vi "Report.vi"() -> ()   [LabVIEW 2017]
uses:
  <vilib>/Utility/miscctls.llb/LVRowAndColumnUnsignedTypeDef.ctl
  bcf87072-937c-4590-92ea-1cc62e0fba93.vi
  a160b8e7-0040-4e34-a052-5f80b3aab475.vi
  <vilib>/Array/Sort 2D Array - Pop Stack.vi
  <vilib>/Array/Sort 2D Array - Push Stack.vi
  <vilib>/addons/database/Connection.llb/DB Tools Open Connec (String).vi
  <vilib>/addons/database/Auxilliary.llb/DB Tools Format Datetime String (Time Stamp).vi
  <vilib>/Utility/file.llb/Write Delimited Spreadsheet (string).vi
  Global/Global 1.vi
  <vilib>/regexp/Match Regular Expression.xnode
  <vilib>/addons/database/NI_Database_API.lvlib
  <vilib>/Utility/NIReport.llb/NI_report.lvclass
  <vilib>/Utility/NIReport.llb/Append Text Table to Report (wrap).vi
panel:
  out "to date/time":string
  out "from date/time":string
  out "reposr save header":string[](array[string])
  in  "SELECT REPORT TYPE":string(combo)="WITH TRECIABILITY"
  out "error out":errorcluster
  in  "error in (no error)":errorcluster
  in  "GET REPORT":bool
  in  "EXIT":bool
  in  "EXPORT TO EXCEL":bool
  in  "TO":timestamp format="%<%x>T"
  in  "FROM":timestamp format="%<%x>T"
  in  "BARCODE":string
  in  "TYPE":string(combo)="DATE TIME"
  in  "STATION WISE":string(combo)="0"
  out "Table":string[][](table)
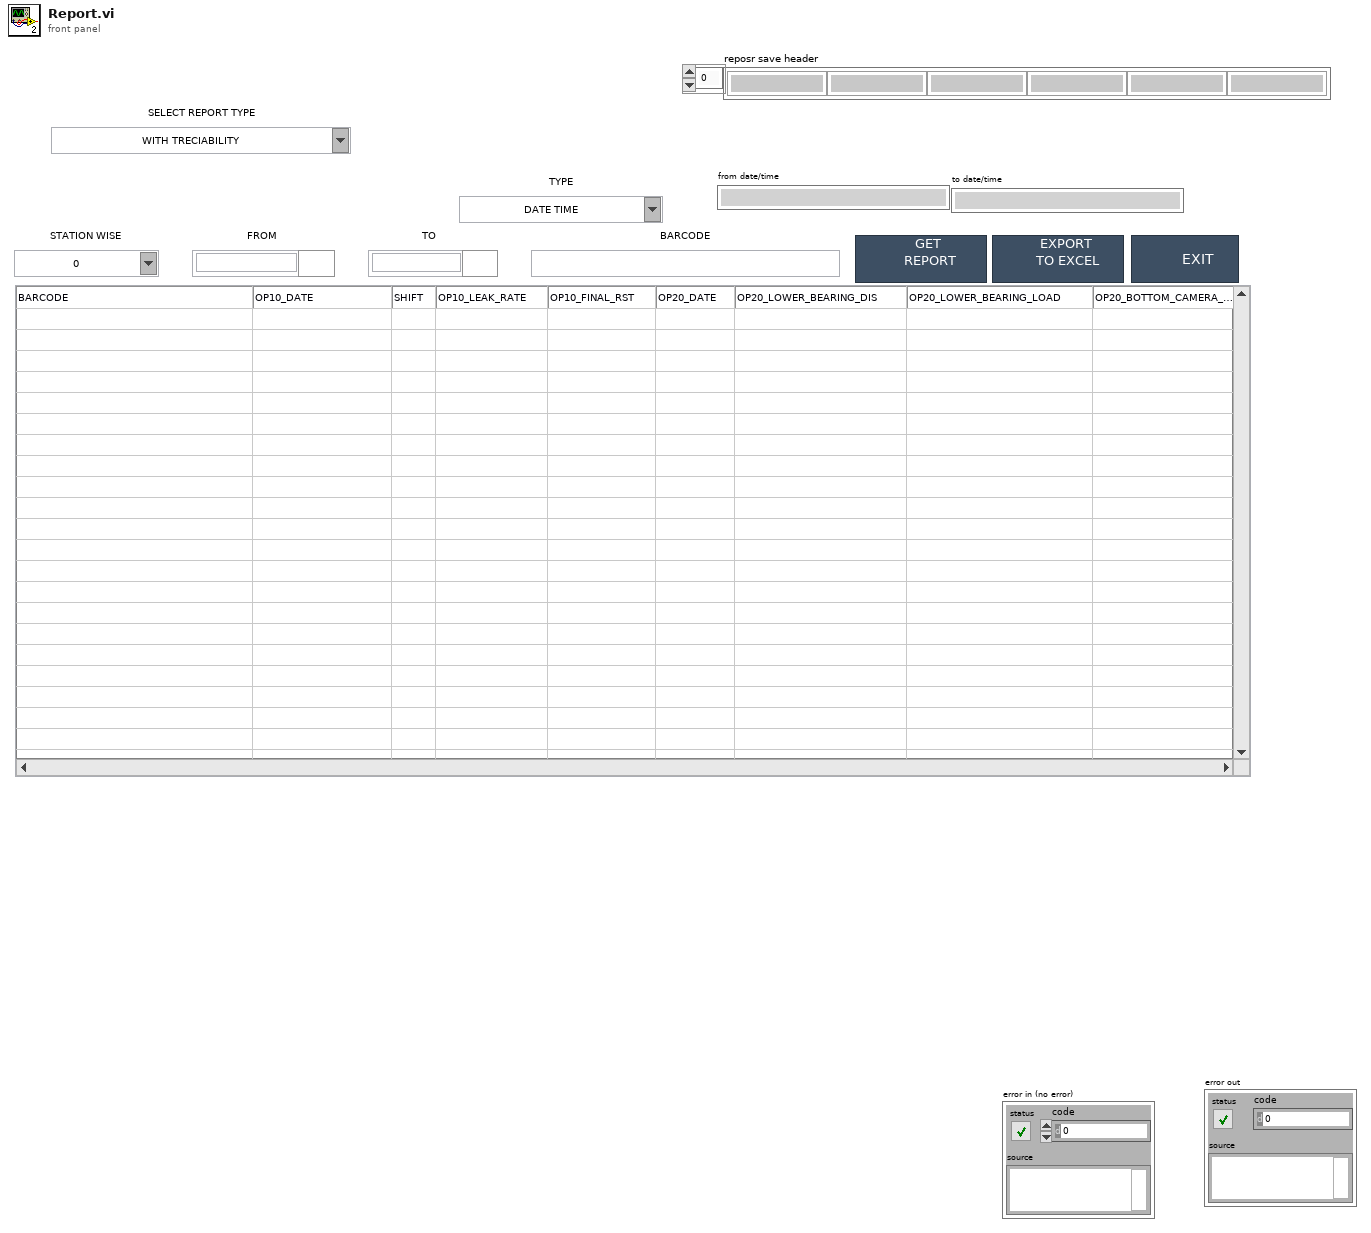
[diagram p1: front panel]
types:
  T1 = typedef "NI_Database_API.lvlib/Conn ObjectReference.ctl" = refnum<k1>
  T2 = typedef "LVRowAndColumnUnsignedTypeDef.ctl" = cluster{"Row":u32, "Column":u32}
  T3 = enum16{"Standard Report", "HTML", "Word", "Excel"}
  T4 = enum16{"maximized", "minimized", "normal", "no change"}
  T5 = typedef "LVRowAndColumnTypeDef.ctl" = cluster{"Row":i32, "Column":i32}
  T6 = enum32{"invalid app kind", "Development System", "Run Time System", "Student Edition", "Embedded LabVIEW", "Evaluation", "Custom"}
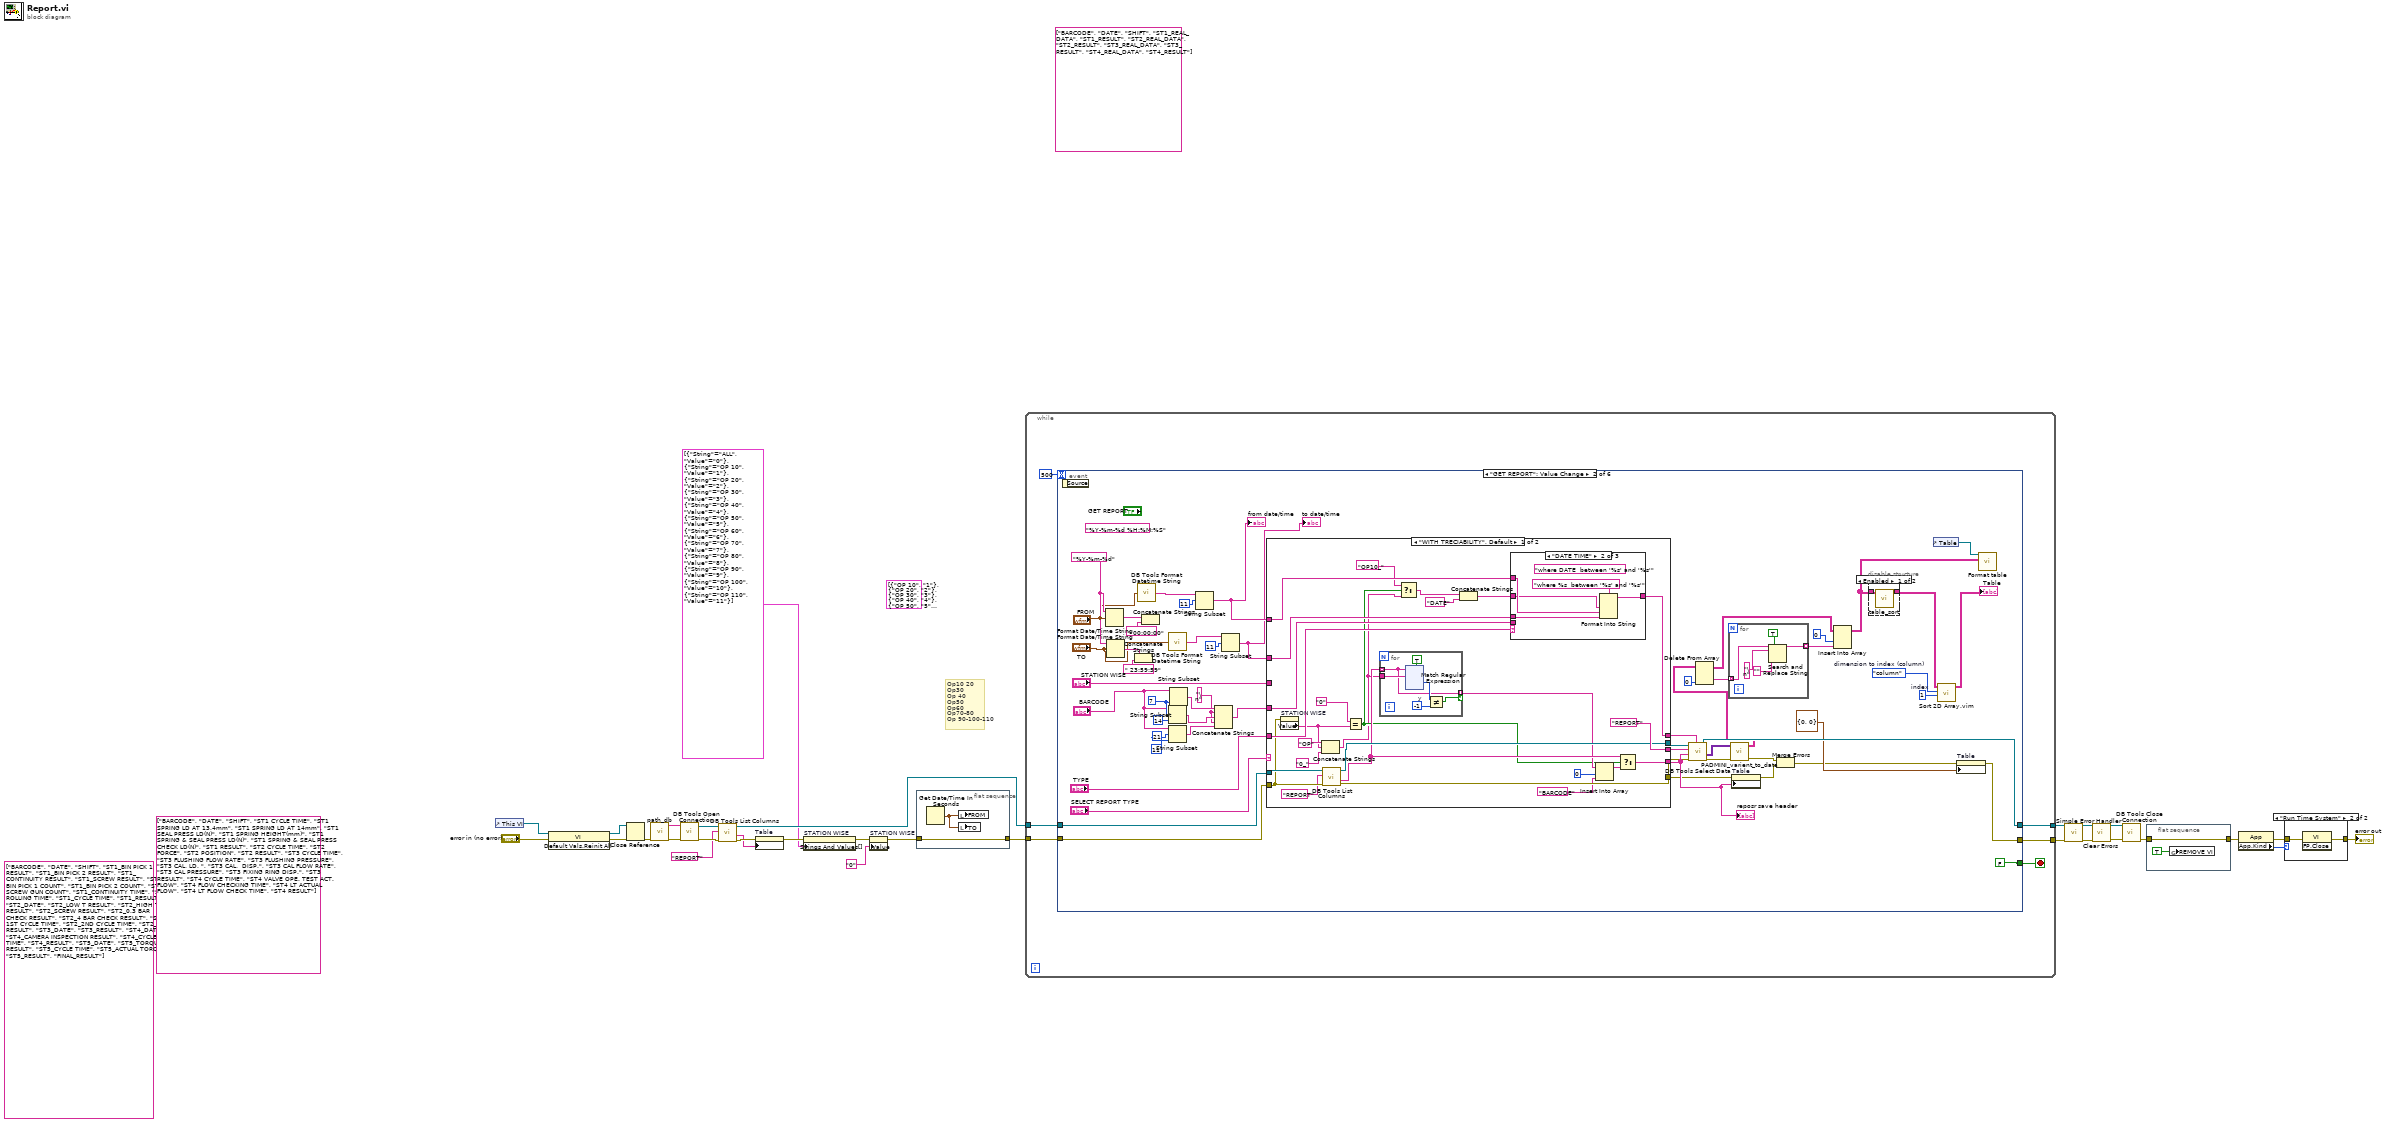
[diagram p0: block diagram]
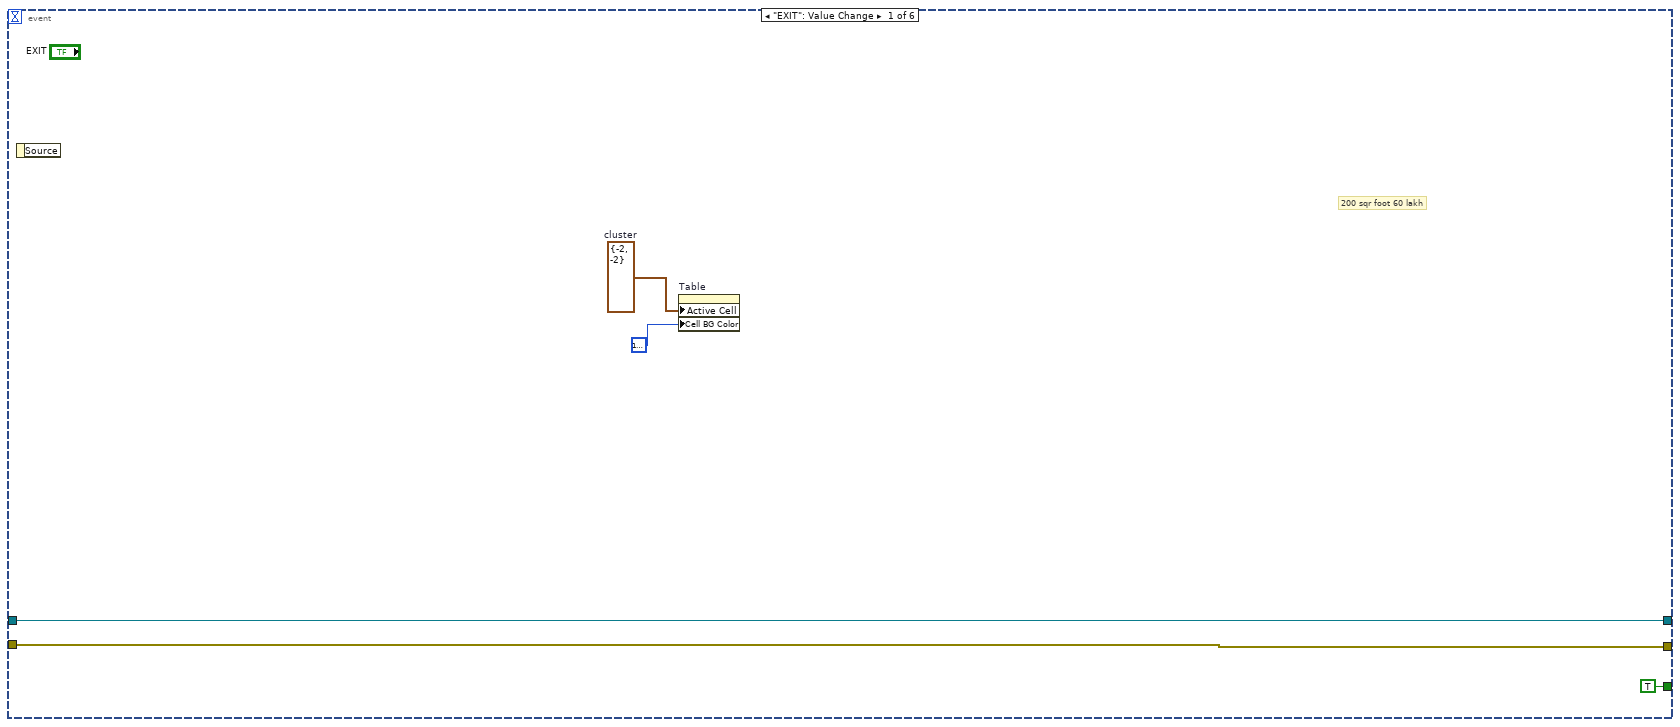
[diagram p2: hidden frame]
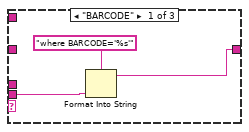
[diagram p4: hidden frame]
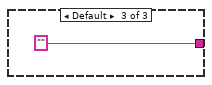
[diagram p5: hidden frame]
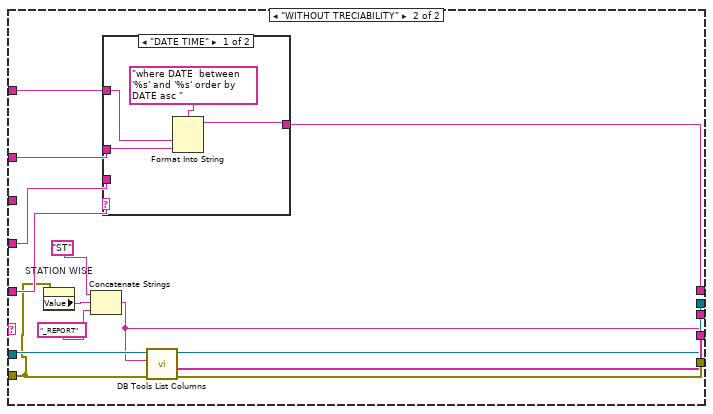
[diagram p6: hidden frame]
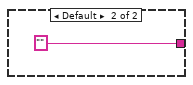
[diagram p7: hidden frame]
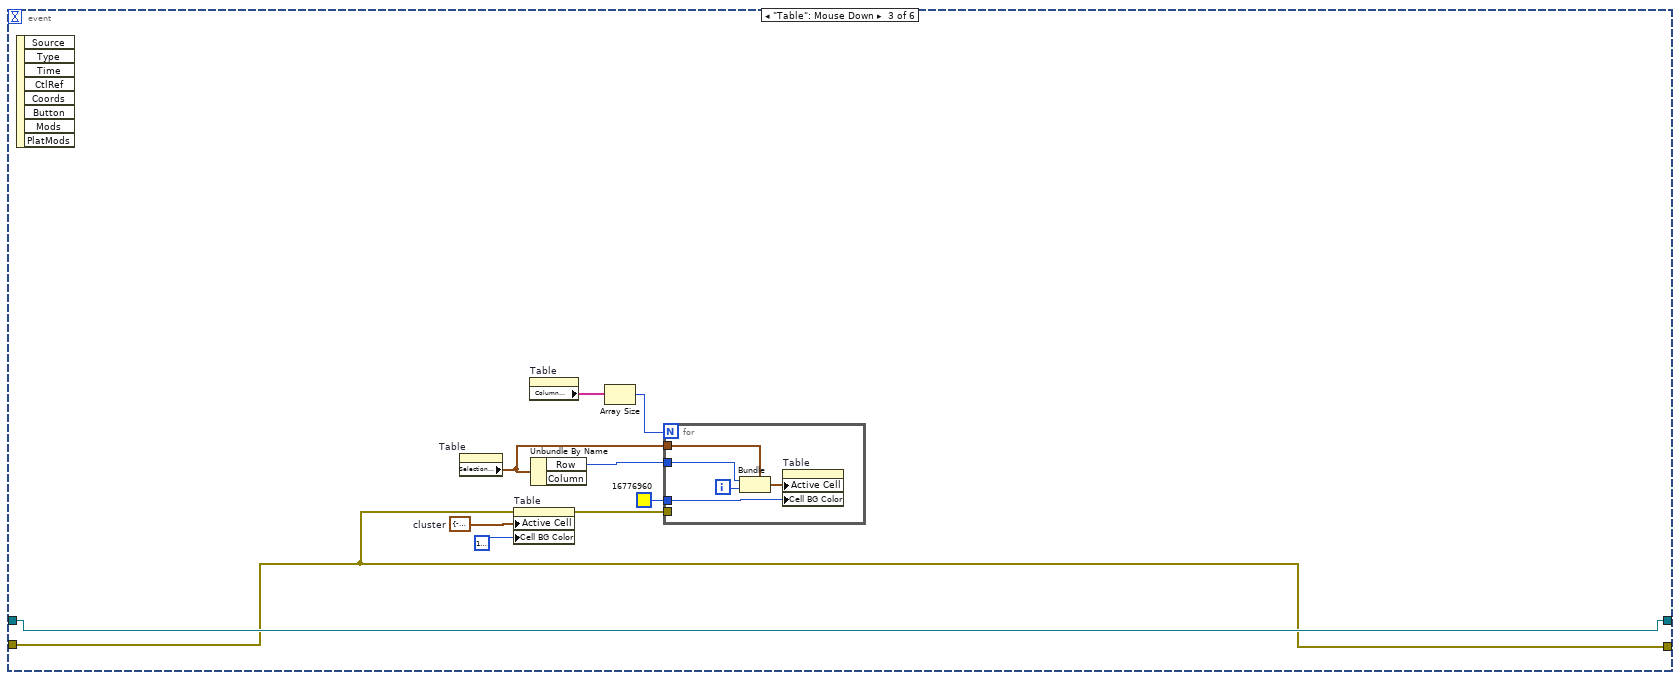
[diagram p8: hidden frame]
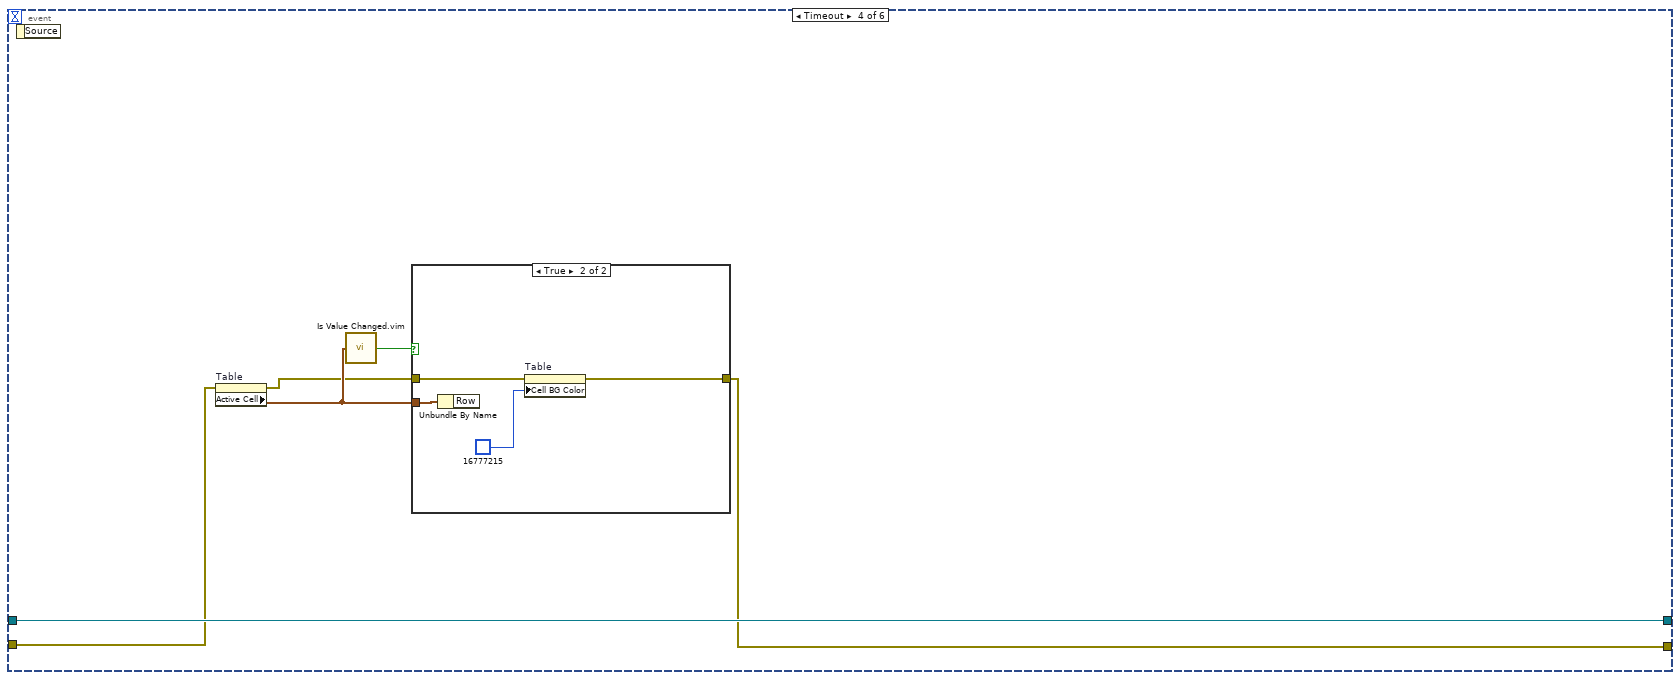
[diagram p9: hidden frame]
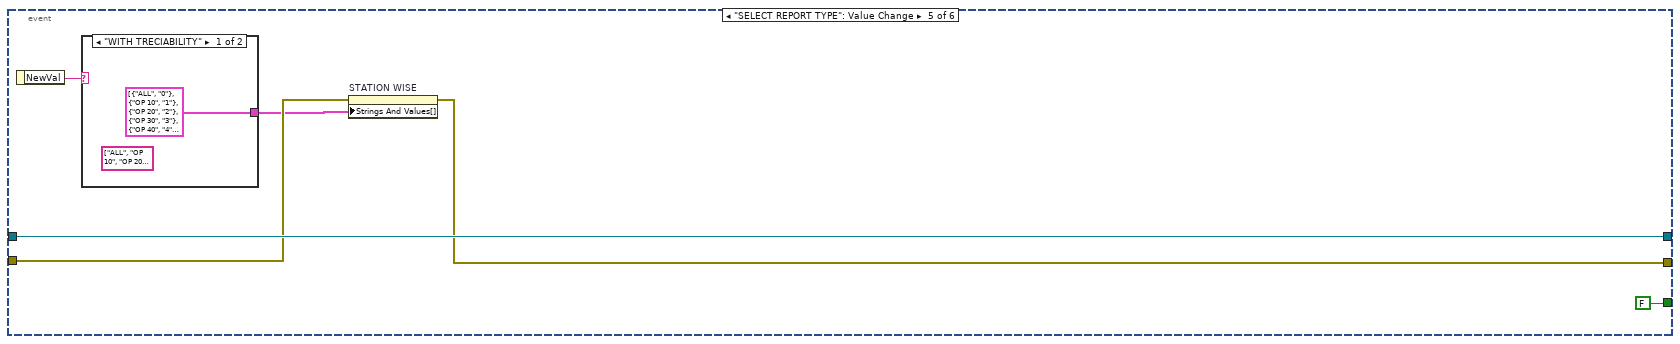
[diagram p11: hidden frame]
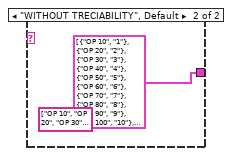
[diagram p12: hidden frame]
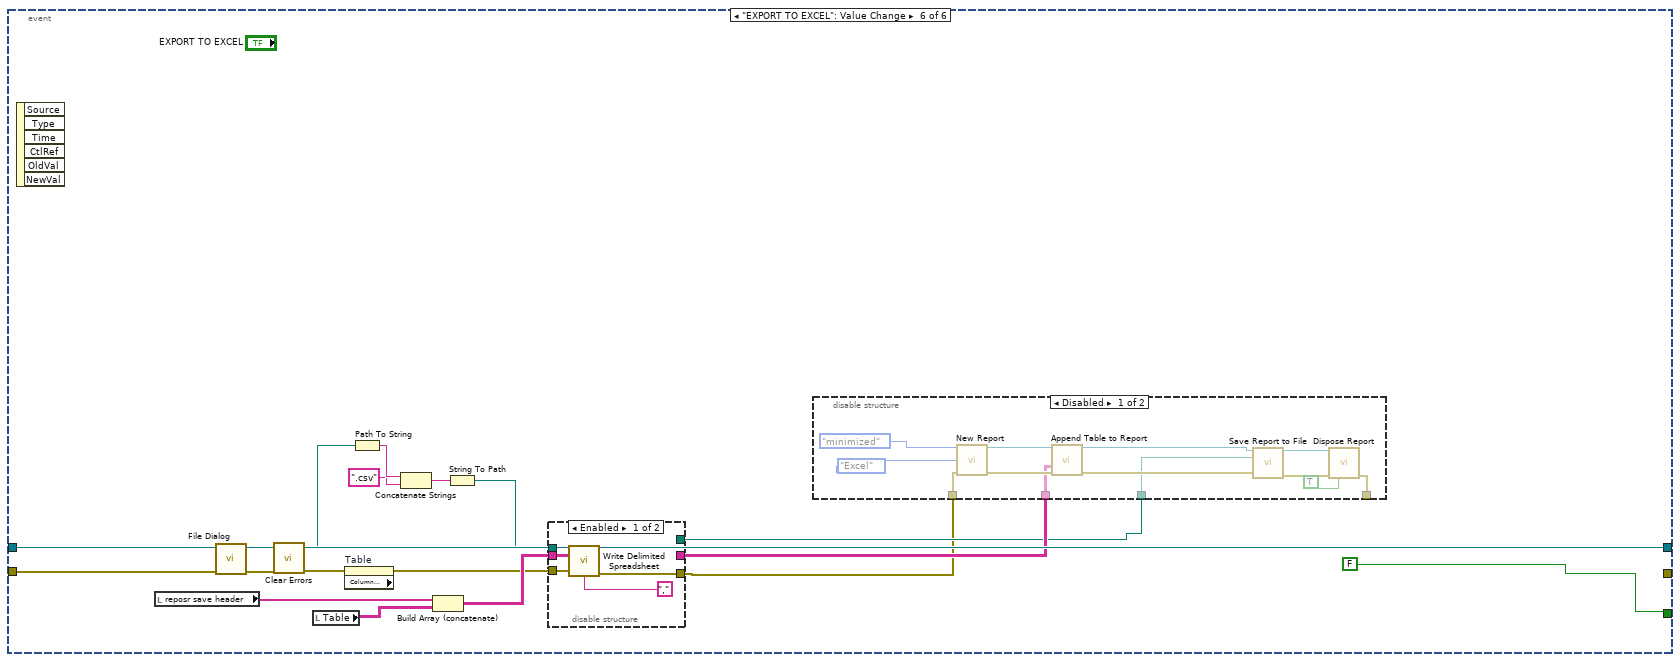
[diagram p13: hidden frame]
diagram:
  (unwired) cluster{"String":string, "Value":string}[] [{"String"="OP 10", "Value"="1"}, {"String"="OP 20", "Value"="2"}, {"String"="OP 30", "Value"="3"}, {"String"="OP 40", "Value"="4"}, {"String"="OP 50", "Value"="5"}, {"String"="OP 60", "Value"="6"}, {"String"="OP 70", "Value"="7"}, {"String"="OP 80", "Value"="8"}, {"String"="OP 90", "Value"="9"}, {"String"="OP 100", "Value"="10"}, {"String"="OP 110", "Value"="11"}] ("Strings And Values [] 2")
  (unwired) string[] ["BARCODE", "DATE", "SHIFT", "ST1_REAL_DATA", "ST1_RESULT", "ST2_REAL_DATA", "ST2_RESULT", "ST3_REAL_DATA", "ST3_RESULT", "ST4_REAL_DATA", "ST4_RESULT"]
  (unwired) string[] ["BARCODE", "DATE", "SHIFT", "ST1_BIN PICK 1 RESULT", "ST1_BIN PICK 2 RESULT", "ST1_CONTINUITY RESULT", "ST1_SCREW RESULT", "ST1_BIN PICK 1 COUNT", "ST1_BIN PICK 2 COUNT", "ST1_SCREW GUN COUNT", "ST1_CONTINUITY TIME", "ST1_ROLLING TIME", "ST1_CYCLE TIME", "ST1_RESULT", "ST2_DATE", "ST2_LOW T RESULT", "ST2_HIGH T RESULT", "ST2_SCREW RESULT", "ST2_0.3 BAR CHECK RESULT", "ST2_4 BAR CHECK RESULT", "ST2_1ST CYCLE TIME", "ST2_2ND CYCLE TIME", "ST2_RESULT", "ST3_DATE", "ST3_RESULT", "ST4_DATE", "ST4_CAMERA INSPECTION RESULT", "ST4_CYCLE TIME", "ST4_RESULT", "ST5_DATE", "ST5_TORQUE RESULT", "ST5_CYCLE TIME", "ST5_ACTUAL TORQUE", "ST5_RESULT", "FINAL_RESULT"]
  (unwired) string[] ["BARCODE", "DATE", "SHIFT", "ST1 CYCLE TIME", "ST1 SPRING LD AT 13.4mm", "ST1 SPRING LD AT 14mm", "ST1 SEAL PRESS LD(N)", "ST1 SPRING HEIGHT(mm)", "ST1 SPRING & SEAL PRESS LD(N)", "ST1 SPRING & SEAL PRESS CHECK LD(N)", "ST1 RESULT", "ST2 CYCLE TIME", "ST2 FORCE", "ST2 POSITION", "ST2 RESULT", "ST3 CYCLE TIME", "ST3 FLUSHING FLOW RATE", "ST3 FLUSHING PRESSURE", "ST3 CAL. LD. ", "ST3 CAL.  DISP.", "ST3 CAL FLOW RATE", "ST3 CAL PRESSURE", "ST3 FIXING RING DISP.", "ST3 RESULT", "ST4 CYCLE TIME", "ST4 VALVE OPE. TEST ACT. FLOW", "ST4 FLOW CHECKING TIME", "ST4 LT ACTUAL FLOW", "ST4 LT FLOW CHECK TIME", "ST4 RESULT"]
  # "Op10 20\nOp30\nOp 40\nOp50\nOp60\nOp70-80\nOp 90-100-110"
  n1 = control-ref of="This VI"() -> (w28:refnum<vi>)
  n2 = invoke class="VI" method="Default Vals.Reinit All"(reference=w28, error in="error in (no error)") -> (reference out=w26:refnum<vi>, error out=w25:errorcluster)  [unwired: 1 in, 1 out]
  n3 = Close Reference(reference=w26, error in (no error)=w25) -> (error out=w16:errorcluster)
  n4 = call "path_db.vi"("error in"=w16) -> ("error out"=w18:errorcluster, "resulting string"=w17:string)  [unwired: 9 in]
  n5 = call-poly <vilib>:"DB Tools Open Connection.vi"("error in (no error)"=w18, "connection information"=w17) -> ("error out"=w11:errorcluster, "connection reference"=w8:T1)  [unwired: 6 in]
  n6 = call <vilib>:"DB Tools List Columns.vi"("error in (no error)"=w11, "table"="REPORT", "connection reference"=w8) -> ("error out"=w10:errorcluster, "columns"=w7:string[], "connection reference out"=w9:T1)  [unwired: 1 in, 1 out]
  n7 = property on="Table" class="Tbl (strict)"(error in=w10, "Column Headers[]"=w7) -> (error out=w13:errorcluster)  [unwired: 1 in, 1 out]
  n8 = property on="STATION WISE" class="CmbBox"(error in=w13, "Strings And Values[]"=cluster{"String":string, "Value":string}[] [{"String"="ALL", "Value"="0"}, {"String"="OP 10", "Value"="1"}, {"String"="OP 20", "Value"="2"}, {"String"="OP 30", "Value"="3"}, {"String"="OP 40", "Value"="4"}, {"String"="OP 50", "Value"="5"}, {"String"="OP 60", "Value"="6"}, {"String"="OP 70", "Value"="7"}, {"String"="OP 80", "Value"="8"}, {"String"="OP 90", "Value"="9"}, {"String"="OP 100", "Value"="10"}, {"String"="OP 110", "Value"="11"}] ("Strings And Values [] 2")) -> (error out=w5:errorcluster)  [unwired: 1 in, 1 out]
  n9 = property on="STATION WISE" class="CmbBox"(error in=w5, "Value"="0") -> (error out=w4:errorcluster)  [unwired: 1 in, 1 out]
  n10 = flat-sequence {
    tunnel: w4 -> [w29]
    tunnel: [w29] -> w12
    frame #0 {
      n11 = Get Date/Time In Seconds() -> (seconds since 1Jan1904=w30:timestamp)
      n12 = local write "FROM"(w30) -> ()
      n13 = local write "TO"(w30) -> ()
    }
  }
  n14 = while {
    tunnel: [w33] -> w1
    tunnel: w12 -> [w35]
    tunnel: w9 -> [w34]
    tunnel: [w32] -> w14
    stop <- w36 stop-if-true
    n15 = event shown="[1] \"GET REPORT\": Value Change" {
      selector: _ -> [_ _ _ _ _ _]
      dyn-events: _ -> [_ _ _ _ _ _]
      timeout: 500 -> [_ _ _ _ _ _]
      tunnel: [TRUE FALSE _ _ FALSE FALSE] -> w36
      tunnel: w35 -> [w39 w79 w287 w296 w308 w317]
      tunnel: w34 -> [w40 w77 w288 w299 w310 w328]
      tunnel: [w40 w85 w288 w299 w310 w328] -> w32
      tunnel: [w39 w67 w287 w294 w305 _] -> w33
      event "EXIT": Value Change {
        w37 = cluster{"Row":i32, "Row":i32} {"Row"=-2, "Row"=-2}  # cluster
        # "200 sqr foot 60 lakh"
        n16 = event-data() -> ()  [unwired: 1 in, 1 out]
        n17 = property on="Table" class="Tbl (strict)"("Active Cell"=w37, "Cell BG Color"=u32 16777226) -> ()  [unwired: 2 in, 2 out]
      }
      event "GET REPORT": Value Change {
        w55 = 1  # index
        w56 = enum16{"column", "row"}."column"  # dimension to index (column)
        w59 = "\n"
        w66 = 7 ("line index")
        (unwired) "%Y-%m-%d %H:%M:%S" ("time format string (%c)")
        w93 = "%Y-%m-%d" ("time format string (%c)")
        n18 = event-data() -> ()  [unwired: 1 in, 1 out]
        n19 = Format Date/Time String(time format string (%c)=w93, seconds (now)="FROM") -> (date/time string=w89:string)  [unwired: 1 in]
        n20 = Format Date/Time String(time format string (%c)=w93, seconds (now)="TO") -> (date/time string=w87:string)  [unwired: 1 in]
        n21 = Concatenate Strings(w87, " 23:59:59" ("time format string (%c)")) -> ()  [unwired: 1 out]
        n22 = call-poly <vilib>:"DB Tools Format Datetime String.vi"("time stamp"="FROM") -> ("date/time string"=w49:string)
        n23 = Concatenate Strings(w89, " 00:00:00" ("time format string (%c)")) -> ()  [unwired: 1 out]
        n24 = call-poly <vilib>:"DB Tools Format Datetime String.vi"("time stamp"="TO") -> ("date/time string"=w46:string)
        n25 = String Subset(string="BARCODE", offset (0)=w66, length (rest)=14 ("line index")) -> (substring=w61:string)
        n26 = String Subset(string="BARCODE", offset (0)=21 ("line index"), length (rest)=11 ("line index")) -> (substring=w60:string)
        n27 = String Subset(string="BARCODE", length (rest)=w66) -> (substring=w62:string)  [unwired: 1 in]
        n28 = String Subset(string=w49, offset (0)=11) -> (substring=w48:string)  [unwired: 1 in]
        "from date/time" <- w48
        n29 = Concatenate Strings(w62, w59, w61, w59, w60) -> (w58:string)
        n30 = String Subset(string=w46, offset (0)=11) -> (substring=w45:string)  [unwired: 1 in]
        "to date/time" <- w45
        n31 = case shown="\"WITH TRECIABILITY\", Default" "SELECT REPORT TYPE" {
          tunnel: "TYPE" -> [w130 w273]
          tunnel: [w129 w272] -> w94
          tunnel: w58 -> [w128 w271]
          tunnel: w48 -> [w127 w270]
          tunnel: w45 -> [w112 w266]
          tunnel: "STATION WISE" -> [_ _]
          tunnel: ["REPORT" w261] -> w80
          tunnel: w79 -> [w118 w260]
          tunnel: [w123 w265] -> w74
          tunnel: [w110 w264] -> w78
          tunnel: w77 -> [w125 w263]
          tunnel: [w124 w262] -> w76
          frame "WITH TRECIABILITY", Default {
            n32 = property on="STATION WISE" class="CmbBox"(error in=w118) -> ("Value"=w113:string)  [unwired: 1 in, 2 out]
            n33 = Concatenate Strings("OP" ("element"), w113, "0_" ("element")) -> (w105:string)
            n34 = call <vilib>:"DB Tools List Columns.vi"("error in (no error)"=w118, "table"="REPORT", "connection reference"=w125) -> ("error out"=w123:errorcluster, "columns"=w117:string[], "connection reference out"=w124:T1)  [unwired: 1 in, 1 out]
            n35 = Equal?(x="0", y=w113) -> (x = y?=w107:bool)
            n36 = for {
              tunnel: w117 -> [w132] mode=indexing
              tunnel: w105 -> [w136]
              tunnel: [w132] -> w111 mode=indexing if=w131
              w133 = -1  # y
              n37 = xnode "Match Regular Expression"("input string"=w132, "regular expression"=w136, "multiline? (F)"=TRUE) -> ("offset past match"=w134:i32)  [unwired: 3 in, 4 out]
              n38 = Not Equal?(x=w134, y=w133) -> (x != y?=w131:bool)
            }
            n39 = Select(t="OP10_", s=w107, f=w105) -> (s? t:f=w104:string)
            n40 = Concatenate Strings(w104, "DATE") -> (w108:string)
            n41 = case shown="\"DATE TIME\"" w130 {
              tunnel: [w252 w257 ""] -> w129
              tunnel: w128 -> [w251 _ _]
              tunnel: w127 -> [_ w256 _]
              tunnel: w112 -> [_ w255 _]
              tunnel: w108 -> [_ w254 _]
              frame "BARCODE" {
                n42 = Format Into String(format string="where BARCODE='%s'", w251) -> (resulting string=w252:string)  [unwired: 2 in, 1 out]
              }
              frame "DATE TIME" {
                (unwired) "where DATE  between '%s' and '%s'"
                n43 = Format Into String(format string="where %s  between '%s' and '%s'", w254, w256, w255) -> (resulting string=w257:string)  [unwired: 2 in, 1 out]
              }
              frame Default {
              }
            }
            n44 = Insert Into Array(array=w111, index=0, new element="BARCODE" ("String")) -> (w121:string[])
            n45 = Select(t=w117, s=w107, f=w121) -> (s? t:f=w110:string[])
          }
          frame "WITHOUT TRECIABILITY" {
            n46 = property on="STATION WISE" class="CmbBox"(error in=w260) -> ("Value"=w269:string)  [unwired: 1 in, 2 out]
            n47 = Concatenate Strings("ST", w269, "_REPORT") -> (w261:string)
            n48 = case shown="\"DATE TIME\"" w273 {
              tunnel: [w277 ""] -> w272
              tunnel: w271 -> [_ _]
              tunnel: w270 -> [w276 _]
              tunnel: w266 -> [w275 _]
              frame "DATE TIME" {
                n49 = Format Into String(format string="where DATE  between '%s' and '%s' order by DATE asc ", w276, w275) -> (resulting string=w277:string)  [unwired: 2 in, 1 out]
              }
              frame Default {
              }
            }
            n50 = call <vilib>:"DB Tools List Columns.vi"("error in (no error)"=w260, "table"=w261, "connection reference"=w263) -> ("error out"=w265:errorcluster, "columns"=w264:string[], "connection reference out"=w262:T1)  [unwired: 1 in, 1 out]
          }
        }
        "reposr save header" <- w78
        n51 = call <vilib>:"DB Tools Select Data.vi"("condition"=w94, "error in (no error)"=w74, "columns"=w78, "table"=w80, "connection reference"=w76) -> ("error out"=w83:errorcluster, "data"=w86:variant[][], "connection reference out"=w85:T1)  [unwired: 1 in]
        n52 = call "PADMINI_varient_to_data.vi"("error in (no error)"=w83, "data"=w86) -> ("error out"=w81:errorcluster, "Array"=w69:string[][])  [unwired: 8 in]
        n53 = Delete From Array(array=w69, index (col)=0 ("disabled index (col)")) -> (deleted portion=w72:string[], array with subset deleted=w70:string[][])  [unwired: 2 in]
        n54 = for {
          tunnel: w72 -> [w100] mode=indexing
          tunnel: [w99] -> w71 mode=indexing
          n55 = Search and Replace String(replace all?=TRUE ("replace all? (F)"), input string=w100, search string="\n", replace string="" ("replace string (\"\")")) -> (result string=w99:string)  [unwired: 4 in, 3 out]
        }
        n56 = property on="Table" class="Tbl (strict)"(error in=w74, "Column Headers[]"=w78) -> (error out=w82:errorcluster)  [unwired: 1 in, 1 out]
        n57 = Merge Errors(w81, w82) -> (w53:errorcluster)
        n58 = Insert Into Array(array=w70, index (col)=0 ("disabled index (col)"), new element=w71) -> (w44:string[][])  [unwired: 1 in]
        n59 = disable-structure shown="Enabled" {
          disable-tunnel: w44 -> [w97 w98]
          disable-tunnel: [w96 w98] -> w43
          frame Enabled {
            n60 = call "table_sort.vi"("Table in"=w97) -> ("Table"=w96:string[][])  [unwired: 9 in]
          }
          frame Disabled {
          }
        }
        n61 = control-ref of="Table"() -> (w54:refnum<vi>)
        n62 = call "Sort 2D Array.vim"("index"=w55, "dimension to index (column)"=w56, "2D array"=w43) -> ("sorted 2D array"=→"Table":string[][])  [unwired: 7 in, 1 out]
        n63 = property on="Table" class="Tbl (strict)"(error in=w53, "Index Values"=T2 {"Row"=0, "Column"=0}) -> (error out=w67:errorcluster)  [unwired: 1 in, 1 out]
        n64 = call "Format table.vi"("Table Control"=w44, "reference"=w54) -> ()  [unwired: 7 in, 1 out]
      }
      event "Table": Mouse Down {
        w282 = cluster{"Row":i32, "Row":i32} {"Row"=-2, "Row"=-2}  # cluster
        n65 = event-data() -> ()  [unwired: 1 in, 8 out]
        n66 = property on="Table" class="Tbl (strict)"() -> ("Selection Start"=w284:T5)  [unwired: 2 in, 2 out]
        n67 = property on="Table" class="Tbl (strict)"(error in=w287, "Active Cell"=w282, "Cell BG Color"=u32 16777226) -> (error out=w283:errorcluster)  [unwired: 1 in, 1 out]
        n68 = property on="Table" class="Tbl (strict)"() -> ("Column Headers[]"=w280:string[])  [unwired: 2 in, 2 out]
        n69 = Unbundle By Name(w284) -> ("Row"=w286:i32)  [unwired: 1 out]
        n70 = Array Size(array=w280) -> (size(s)=w279:i32)
        n71 = for {
          N: w279 -> [_]
          tunnel: u32 16776960 -> [w293]
          tunnel: w284 -> [w292]
          tunnel: w286 -> [w291]
          tunnel: w283 -> [_]
          i -> [w290]
          n72 = Bundle(cluster=w292, "Row"=w291, "Column"=w290) -> (w289:T5)
          n73 = property on="Table" class="Tbl (strict)"("Active Cell"=w289, "Cell BG Color"=w293) -> ()  [unwired: 2 in, 2 out]
        }
      }
      event Timeout {
        n74 = event-data() -> ()  [unwired: 1 in, 1 out]
        n75 = property on="Table" class="Tbl (strict)"(error in=w296) -> (error out=w295:errorcluster, "Active Cell"=w298:T5)  [unwired: 1 in, 1 out]
        n76 = call "Is Value Changed.vim"("value"=w298) -> ("changed or first call?"=w297:bool)
        n77 = case shown="True" w297 {
          tunnel: w298 -> [_ w304]
          tunnel: w295 -> [w300 w302]
          tunnel: [w300 w301] -> w294
          frame False {
          }
          frame True {
            n78 = Unbundle By Name(w304) -> ()  [unwired: 1 out]
            n79 = property on="Table" class="Tbl (strict)"(error in=w302, "Cell BG Color"=u32 16777215) -> (error out=w301:errorcluster)  [unwired: 1 in, 1 out]
          }
        }
      }
      event "SELECT REPORT TYPE": Value Change {
        n80 = event-data() -> ("NewVal"=w309:string)  [unwired: 1 in]
        n81 = case shown="\"WITH TRECIABILITY\"" w309 {
          tunnel: [cluster{"String":string, "Value":string}[] [{"String"="ALL", "Value"="0"}, {"String"="OP 10", "Value"="1"}, {"String"="OP 20", "Value"="2"}, {"String"="OP 30", "Value"="3"}, {"String"="OP 40", "Value"="4"}, {"String"="OP 50", "Value"="5"}, {"String"="OP 60", "Value"="6"}, {"String"="OP 70", "Value"="7"}, {"String"="OP 80", "Value"="8"}, {"String"="OP 90", "Value"="9"}, {"String"="OP 100", "Value"="10"}, {"String"="OP 110", "Value"="11"}] ("Strings And Values [] 2") cluster{"String":string, "Value":string}[] [{"String"="OP 10", "Value"="1"}, {"String"="OP 20", "Value"="2"}, {"String"="OP 30", "Value"="3"}, {"String"="OP 40", "Value"="4"}, {"String"="OP 50", "Value"="5"}, {"String"="OP 60", "Value"="6"}, {"String"="OP 70", "Value"="7"}, {"String"="OP 80", "Value"="8"}, {"String"="OP 90", "Value"="9"}, {"String"="OP 100", "Value"="10"}, {"String"="OP 110", "Value"="11"}] ("Strings And Values [] 2")] -> w306
          frame "WITH TRECIABILITY" {
            (unwired) string[] ["ALL", "OP 10", "OP 20", "OP 30", "OP 40", "OP 50", "OP 60", "OP 70", "OP 80", "OP 90", "OP 100", "OP 110"] ("Strings []")
          }
          frame "WITHOUT TRECIABILITY", Default {
            (unwired) string[] ["OP 10", "OP 20", "OP 30", "OP 40", "OP 50", "OP 60", "OP 70", "OP 80", "OP 90", "OP 100", "OP 110"] ("Strings []")
          }
        }
        n82 = property on="STATION WISE" class="CmbBox"(error in=w308, "Strings And Values[]"=w306) -> (error out=w305:errorcluster)  [unwired: 1 in, 1 out]
      }
      event "EXPORT TO EXCEL": Value Change {
        n83 = event-data() -> ()  [unwired: 1 in, 6 out]
        n84 = local read "reposr save header"() -> (w313:string[])
        n85 = call "File Dialog"("error in"=w317) -> ("selected path"=w326:path, "error out"=w327:errorcluster)  [unwired: 11 in, 2 out]
        n86 = call <vilib>:"Clear Errors.vi"("error in (no error)"=w327) -> ("error out"=w320:errorcluster)  [unwired: 5 in, 1 out]
        n87 = local read "Table"() -> (w329:string[][])
        n88 = property on="Table" class="Tbl (strict)" props=["Column Headers[]"](error in=w320) -> (error out=w319:errorcluster)  [unwired: 1 in, 2 out]
        n89 = Path To String(path=w326) -> (string=w325:string)
        n90 = Concatenate Strings(w325, ".csv" ("string")) -> (w323:string)
        n91 = Build Array (concatenate)(w313, w329) -> (w321:string[][])
        n92 = String To Path(string=w323) -> (path=w322:path)
        n93 = disable-structure shown="Enabled" {
          disable-tunnel: w322 -> [w348 w349]
          disable-tunnel: [w347 w351] -> w314
          disable-tunnel: w321 -> [w346 w350]
          disable-tunnel: w319 -> [w344 w351]
          disable-tunnel: [_ w350] -> w316
          disable-tunnel: [_ w349] -> w315
          frame Enabled {
            n94 = call-poly <vilib>:"Write Delimited Spreadsheet.vi"("file path (dialog if empty)"=w348, "2D data"=w346, "error in (no error)"=w344, "delimiter (\\t)"="," ("delimiter (\\t)")) -> ("error out"=w347:errorcluster)  [unwired: 10 in, 1 out]
          }
          frame Disabled {
          }
        }
        n95 = disable-structure shown="Disabled" {
          disable-tunnel: w316 -> [w333 _]
          disable-tunnel: w315 -> [w332 _]
          disable-tunnel: [w331 w343] -> _
          disable-tunnel: w314 -> [w330 w343]
          frame Disabled {
            n96 = call <vilib>:"New Report.vi"("window state (normal)"=T4."minimized", "report type"=T3."Excel", "error in (no error)"=w330) -> ("report out"=w340:refnum<class "NI_report.lvclass">, "error out"=w339:errorcluster)  [unwired: 11 in]
            n97 = call-poly <vilib>:"Append Table to Report.vi"("report in"=w340, "text data"=w333, "error in (no error)"=w339) -> ("report out"=w336:refnum<class "NI_report.lvclass">, "error out"=w338:errorcluster)  [unwired: 9 in, 2 out]
            n98 = call-dynamic "Save Report to File.vi"("report in"=w336, "report file path"=w332, "error in (no error)"=w338) -> ("report out"=w335:refnum<class "NI_report.lvclass">, "error out"=w337:errorcluster)  [unwired: 11 in]
            n99 = call-dynamic "Dispose Report.vi"("report in"=w335, "error in (no error)"=w337, "close report? (T)"=TRUE) -> ("error out"=w331:errorcluster)  [unwired: 12 in]
          }
          frame Enabled {
          }
        }
      }
    }
  }
  n100 = call <vilib>:"Simple Error Handler.vi"("error in (no error)"=w1) -> ("error out"=w24:errorcluster)  [unwired: 4 in, 4 out]
  n101 = call <vilib>:"Clear Errors.vi"("error in (no error)"=w24) -> ("error out"=w23:errorcluster)  [unwired: 5 in, 1 out]
  n102 = call <vilib>:"DB Tools Close Connection.vi"("error in (no error)"=w23, "connection reference"=w14) -> ("error out"=w15:errorcluster)  [unwired: 5 in]
  n103 = flat-sequence {
    tunnel: [w353] -> w22
    tunnel: w15 -> [w353]
    frame #0 {
      n104 = global write "Global 1.vi" "REMOVE VI"(TRUE ("REMOVE VI")) -> ()
    }
  }
  n105 = property class="App"(error in=w22) -> (error out=w21:errorcluster, "App.Kind"=w20:T6)  [unwired: 1 in, 1 out]
  n106 = case shown="\"Run Time System\"" w20 {
    tunnel: w21 -> [w354 w356]
    tunnel: [w354 w355] -> w19
    frame "Development System", Default {
    }
    frame "Run Time System" {
      n107 = invoke class="VI" method="FP.Close"(error in=w356) -> (error out=w355:errorcluster)  [unwired: 2 in, 2 out]
    }
  }
  "error out" <- w19
